vi "Ctor Device.vi"(8 "error in (no error)":errorcluster, 11 "Simulated Scope in":refnum<class "Simulated Scope.lvclass">) -> (0 "error out":errorcluster, 3 "Simulated Scope out":refnum<class "Simulated Scope.lvclass">)   [LabVIEW 2020, in "Simulated Scope.lvlib" / "Simulated Scope.lvclass"]
uses:
  Simulated Scope.lvclass
  Ref Data.ctl
  Simulated Scope.lvclass/Simulated Scope.ctl
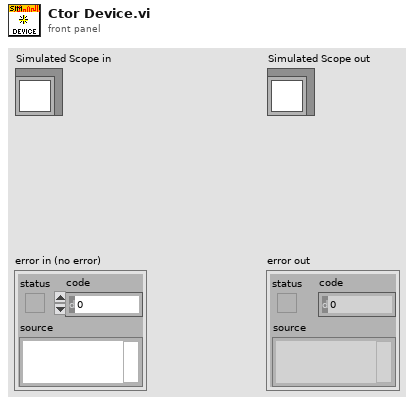
[diagram p1: front panel]
types:
  T1 = typedef "Simulated Scope.lvlib/Simulated Scope.lvclass/Ref Data.ctl" = cluster{"Sim Queue Name":string, "Waveform Queue":refnum<queue>}
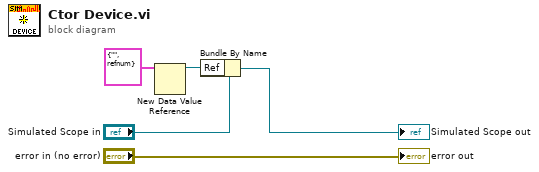
[diagram p0: block diagram]
diagram:
  n1 = New Data Value Reference(data value=T1 {"Sim Queue Name"="", "Waveform Queue"=refnum} ("Ref Data")) -> (data value reference=w1:refnum<data-value>)  [unwired: 1 in, 1 out]
  n2 = Bundle By Name(cluster="Simulated Scope in", "Ref"=w1) -> (→"Simulated Scope out":refnum<class "Simulated Scope.lvclass">)
  "error out" <- "error in (no error)"
